vi "Timer_Call_CountDown_Async.vi"() -> ()   [LabVIEW 2015]
panel:
  out "nombre (de 0 à 1)":dbl
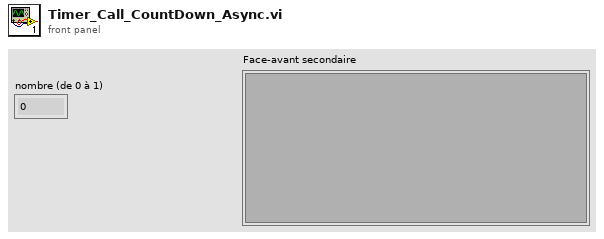
[diagram p1: front panel]
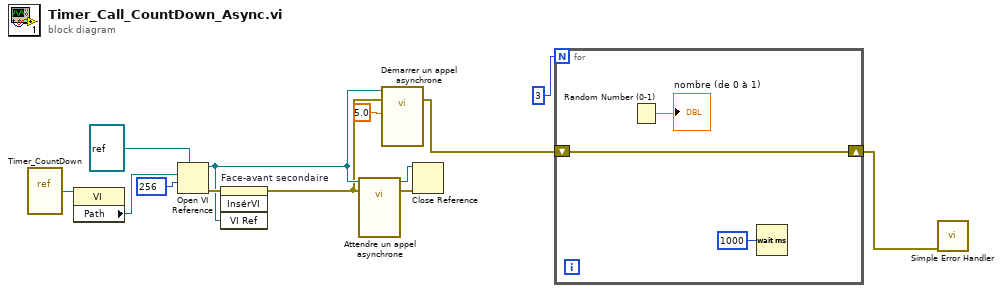
[diagram p0: block diagram]
diagram:
  n1 = vi-ref "Timer_CountDown.vi"() -> (w8:refnum<vi>)
  n2 = property class="VI"(reference=w8) -> ("Path"=w7:path)  [unwired: 1 in, 2 out]
  n3 = Open VI Reference(type specifier VI Refnum (for type only)=refnum<vi> refnum ("spécificateur de type du refnum de VI (pour type seulement)"), vi path=w7, options=256) -> (vi reference=w4:refnum<vi>, error out=w5:errorcluster)  [unwired: 3 in]
  n4 = invoke on="Face-avant secondaire" class="FAsec" method="InsérVI"(error in=w5, "VI Ref"=w4) -> (error out=w1:errorcluster)  [unwired: 2 in, 3 out]
  n5 = call-by-ref "Attendre un appel asynchrone"(reference=w4, error in=w1) -> (reference out=w3:refnum<vi>, error out=w2:errorcluster)  [unwired: 12 in]
  n6 = call-by-ref "Démarrer un appel asynchrone"(reference=w4, error in=w1, "Seconds"=5.0) -> (error out=w9:errorcluster)  [unwired: 11 in, 1 out]
  n7 = Close Reference(reference=w3, error in (no error)=w2) -> ()  [unwired: 1 out]
  n8 = for {
    N: 3 -> [_]
    shift-right: [w15] -> w6
    shift-left: w9 -> [w15]
    n9 = Random Number (0-1)() -> (number: 0 to 1=→"nombre (de 0 à 1)":dbl)
    n10 = Wait (ms)(milliseconds to wait=u32 1000 ("attente (ms)")) -> ()  [unwired: 1 out]
  }
  n11 = call <vilib>:"Simple Error Handler.vi"("error in (no error)"=w6) -> ()  [unwired: 4 in, 5 out]
